vi "AppendConsole.vi"(10 "String":string, 11 "String in":refnum<vi>) -> (1 "console":string, 2 "everything":string, 3 "left over fixed":string)   [LabVIEW 2021]
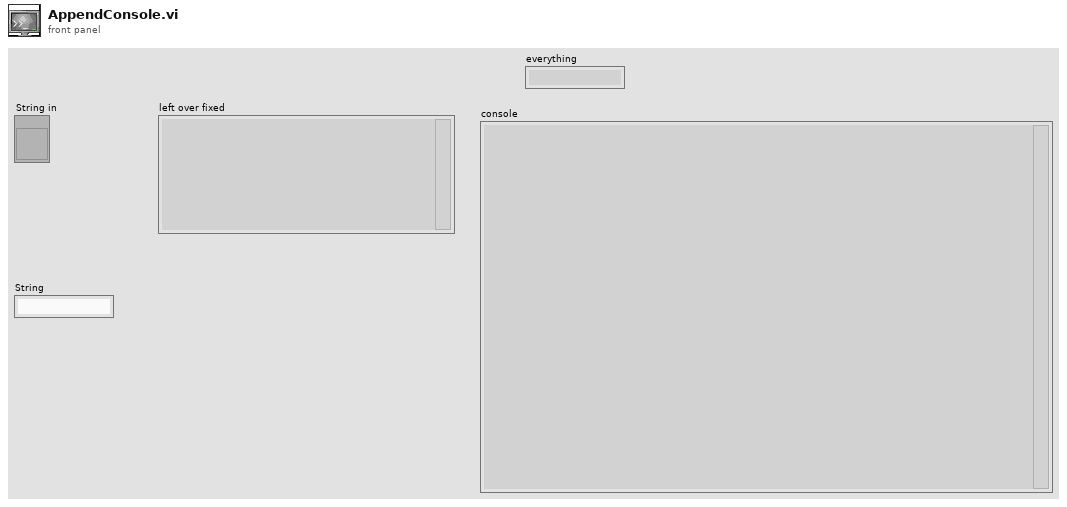
[diagram p1: front panel]
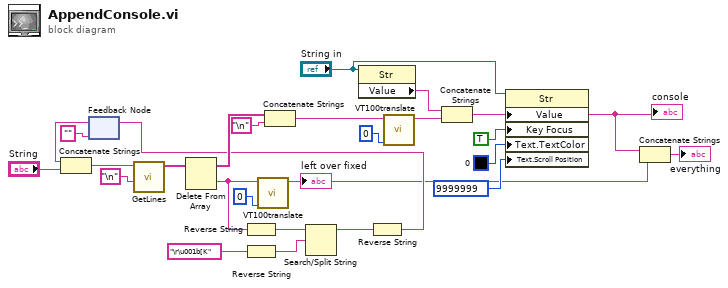
[diagram p0: block diagram]
diagram:
  n1 = feedback #1("" ("Left over raw")) -> (w17:string)
  n2 = Concatenate Strings(w17, "String") -> (w11:string)
  n3 = call "GetLines.vi"("delimiter"="\n", "String"=w11) -> ("Array"=w10:string[])  [unwired: 9 in]
  n4 = Delete From Array(array=w10) -> (deleted portion=w9:string, array with subset deleted=w22:string[])  [unwired: 2 in]
  n5 = Reverse String(1:w9) -> (0:w7:string)
  n6 = Reverse String(1:"\r\u001b[K" ("New Text")) -> (0:w6:string)
  n7 = call "VT100translate.vi"("cursor in"=0, "Text"=w9) -> ("Console fixed"=w2:string)  [unwired: 8 in, 1 out]
  "left over fixed" <- w2
  n8 = Concatenate Strings(w22, "\n" ("regular expression")) -> (w19:string)
  n9 = Search/Split String(string=w7, search string/char (-)=w6) -> (substring before match=w8:string)  [unwired: 1 in, 2 out]
  n10 = property class="Str"(reference="String in") -> ("Value"=w23:string)  [unwired: 1 in, 2 out]
  n11 = Reverse String(1:w8) -> (0:w16:string)
  n12 = feedback-in #1(w16) -> ()
  n13 = call "VT100translate.vi"("cursor in"=0, "Text"=w19) -> ("Console fixed"=w21:string)  [unwired: 8 in, 1 out]
  n14 = Concatenate Strings(w23, w21) -> (w3:string)
  "console" <- w3
  n15 = property on="Property Node" class="Str"(reference="String in", "Value"=w3, "Key Focus"=TRUE, "Text.TextColor"=u32 0 ("Text.Text Colors:Text Color"), "Text.Scroll Position"=u32 9999999) -> ()  [unwired: 1 in, 2 out]
  n16 = Concatenate Strings(w3, w2) -> (→"everything":string)
